vi "触发设置.vi"(6 "Trigger Coupling (0 : DC)":u16(ring) items=["DC", "HF Reject", "LF Reject", "Noise Reject", "AC"], 7 "Trigger Slope (0: Rising)":u16(ring) items=["Rising", "Falling", "Either"], 8 "error in (no error)":errorcluster, 9 "Trigger Level (0.0 V)":dbl, 10 "Trigger Source (0: Channel 1)":u16(ring) items=["Channel 1", "Channel 2", "Channel 3", "Channel 4", "AC Line", "Aux", "Digital Channel 0", "Digital Channel 1", "Digital Channel 2", "Digital Channel 3", "Digital Channel 4", "Digital Channel 5", "Digital Channel 6", "Digital Channel 7", "Digital Channel 8", "Digital Channel 9", "Digital Channel 10", "Digital Channel 11", "Digital Channel 12", "Digital Channel 13", "Digital Channel 14", "Digital Channel 15", "RF"], 11 "VISA resource name":refnum<visa-resource-name>) -> (0 "error out":errorcluster, 3 "VISA resource name out":refnum<visa-resource-name>)   [LabVIEW 2018]
uses:
  Tektronix DPO MSO 2000 4000 Series/Tektronix DPO MSO 2000 4000 Series.lvlib
panel:
  out "输出字符串":string
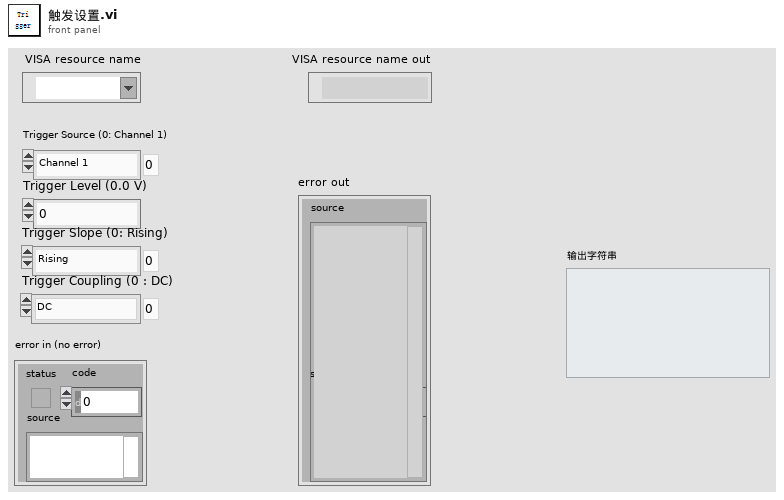
[diagram p1: front panel]
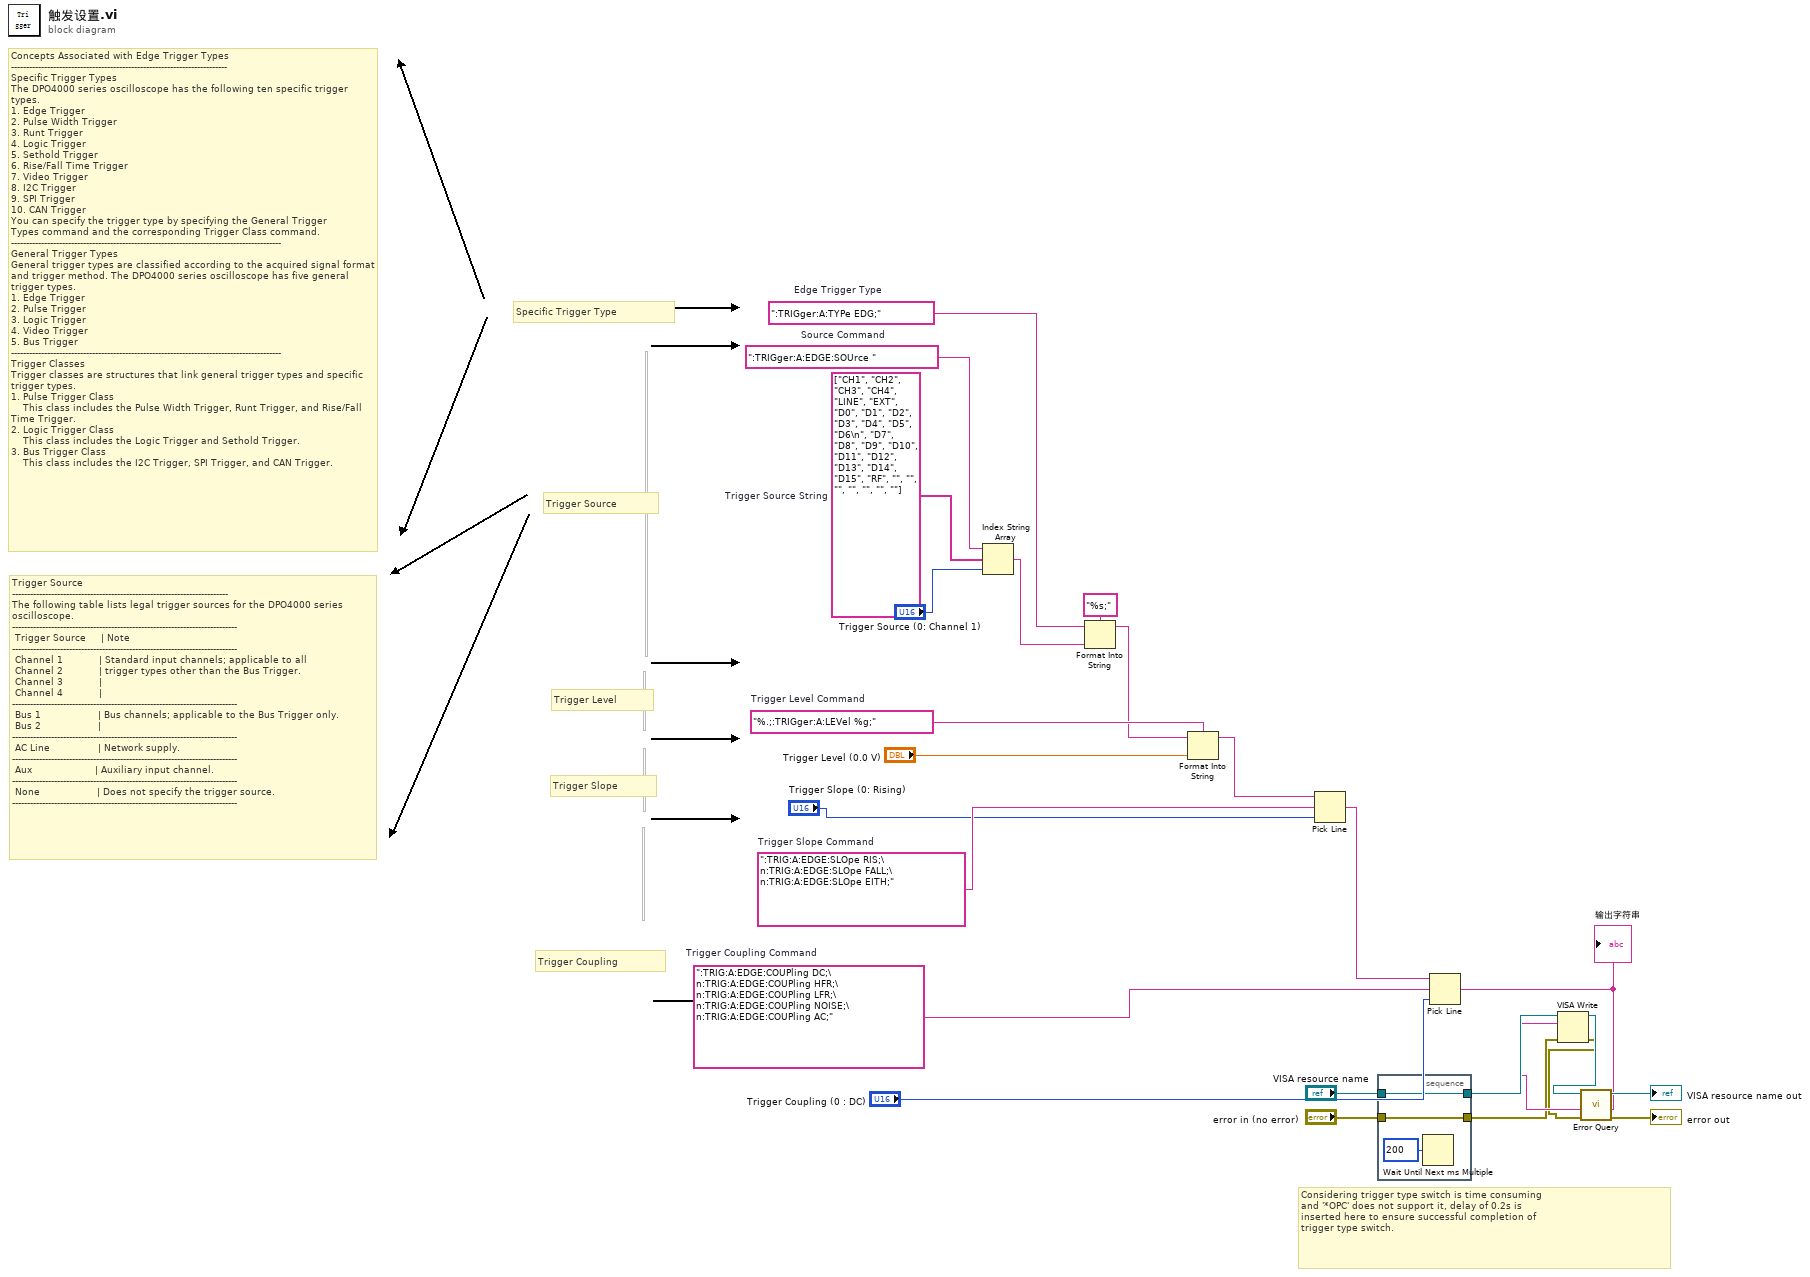
[diagram p0: block diagram]
diagram:
  w12 = ":TRIG:A:EDGE:COUPling DC;\n:TRIG:A:EDGE:COUPling HFR;\n:TRIG:A:EDGE:COUPling LFR;\n:TRIG:A:EDGE:COUPling NOISE;\n:TRIG:A:EDGE:COUPling AC;"  # Trigger Coupling Command
  w18 = string[] ["CH1", "CH2", "CH3", "CH4", "LINE", "EXT", "D0", "D1", "D2", "D3", "D4", "D5", "D6\n", "D7", "D8", "D9", "D10", "D11", "D12", "D13", "D14", "D15", "RF", "", "", "", "", "", "", ""]  # Trigger Source String
  w20 = ":TRIG:A:EDGE:SLOpe RIS;\n:TRIG:A:EDGE:SLOpe FALL;\n:TRIG:A:EDGE:SLOpe EITH;"  # Trigger Slope Command
  w22 = "%.;:TRIGger:A:LEVel %g;"  # Trigger Level Command
  w16 = ":TRIGger:A:TYPe EDG;"  # Edge Trigger Type
  w17 = ":TRIGger:A:EDGE:SOUrce "  # Source Command
  # "Trigger Source\n------------------------------------------------------------------------\nThe following table lists legal trigger sources for the DPO4000 series oscilloscope.\n---------------------------------------------------------------------------\n Trigger Source     | Note                                                           \n---------------------------------------------------------------------------\n Channel 1            | Standard input channels; applicable to all      \n Channel 2            | trigger types other than the Bus Trigger.         \n Channel 3            |     \n Channel 4            |\n---------------------------------------------------------------------------\n Bus 1                   | Bus channels; applicable to the Bus Trigger only.\n Bus 2                   | \n---------------------------------------------------------------------------\n AC Line                | Network supply.\n---------------------------------------------------------------------------\n Aux                     | Auxiliary input channel.\n---------------------------------------------------------------------------\n None                   | Does not specify the trigger source.\n---------------------------------------------------------------------------"
  # "Trigger Coupling"
  # "Trigger Slope"
  # "Trigger Level"
  # "Trigger Source"
  # "Specific Trigger Type"
  # "Concepts Associated with Edge Trigger Types\n------------------------------------------------------------------------\nSpecific Trigger Types\nThe DPO4000 series oscilloscope has the following ten specific trigger types.\n1. Edge Trigger\n2. Pulse Width Trigger\n3. Runt Trigger\n4. Logic Trigger\n5. Sethold Trigger\n6. Rise/Fall Time Trigger\n7. Video Trigger\n8. I2C Trigger\n9. SPI Trigger\n10. CAN Trigger\nYou can specify the trigger type by specifying the General Trigger \nTypes command and the corresponding Trigger Class command.\n------------------------------------------------------------------------------------------\nGeneral Trigger Types \nGeneral trigger types are classified according to the acquired signal format and trigger method. The DPO4000 series oscilloscope has five general trigger types.\n1. Edge Trigger\n2. Pulse Trigger\n3. Logic Trigger\n4. Video Trigger\n5. Bus Trigger\n------------------------------------------------------------------------------------------\nTrigger Classes\nTrigger classes are structures that link general trigger types and specific trigger types.\n1. Pulse Trigger Class\n    This class includes the Pulse Width Trigger, Runt Trigger, and Rise/Fall Time Trigger.\n2. Logic Trigger Class\n    This class includes the Logic Trigger and Sethold Trigger.\n3. Bus Trigger Class\n    This class includes the I2C Trigger, SPI Trigger, and CAN Trigger."
  # "Considering trigger type switch is time consuming\nand '*OPC' does not support it, delay of 0.2s is \ninserted here to ensure successful completion of\ntrigger type switch."
  n1 = Index String Array(1:"Trigger Source (0: Channel 1)", 2:w18, 3:w17) -> (0:w14:string)
  n2 = Format Into String(format string="%s;", initial string=w16, w14) -> (resulting string=w13:string)  [unwired: 1 in, 1 out]
  n3 = Format Into String(format string=w22, initial string=w13, "Trigger Level (0.0 V)") -> (resulting string=w10:string)  [unwired: 1 in, 1 out]
  n4 = Pick Line(string ("")=w10, multi-line string=w20, line index="Trigger Slope (0: Rising)") -> (output string=w9:string)
  n5 = stacked-sequence {
    tunnel: "VISA resource name" -> [w26]
    tunnel: [w26] -> w5
    tunnel: "error in (no error)" -> [w25]
    tunnel: [w25] -> w3
    frame #0 {
      n6 = Wait Until Next ms Multiple(millisecond multiple=u32 200) -> ()  [unwired: 1 out]
    }
  }
  n7 = Pick Line(string ("")=w9, multi-line string=w12, line index="Trigger Coupling (0 : DC)") -> (output string=w4:string)
  "输出字符串" <- w4
  n8 = VISA Write(VISA resource name=w5, write buffer=w4, error in (no error)=w3) -> (VISA resource name out=w2:refnum<visa-resource-name>, error out=w1:errorcluster)  [unwired: 1 out]
  n9 = call "Error Query.vi"("error in (no error)"=w1, "VISA resource name"=w2) -> ("error out"=→"error out":errorcluster, "VISA resource name out"=→"VISA resource name out":refnum<visa-resource-name>)  [unwired: 6 in, 2 out]
